vi "Tutorial_7_ICP_IP_save_table.vi"() -> ()   [LabVIEW 2020]
uses:
  <vilib>/Utility/file.llb/Write Delimited Spreadsheet (string).vi
  <vilib>/Utility/file.llb/Read Delimited Spreadsheet (string).vi
  <vilib>/regexp/Match Regular Expression.xnode
panel:
  out "data out":string
  out "ArraySize":i32
  out "subarray":string[](array[string])
  out "Login Details":string
  out "error out":errorcluster
  in  "file path (dialog if empty)":path
  in  "Registration UI":enum32{"Page 1", "Page 2"}(tab)
  in  "OK Button":bool
  in  "tbl Registration":string[][](table)
  in  "Login UI":enum32{"Page 1"}(tab)
  out "Status":bool
  in  "btnLogin":bool
  in  "Password":string
  in  "User Name":string
  # "Client"
  # "Server"
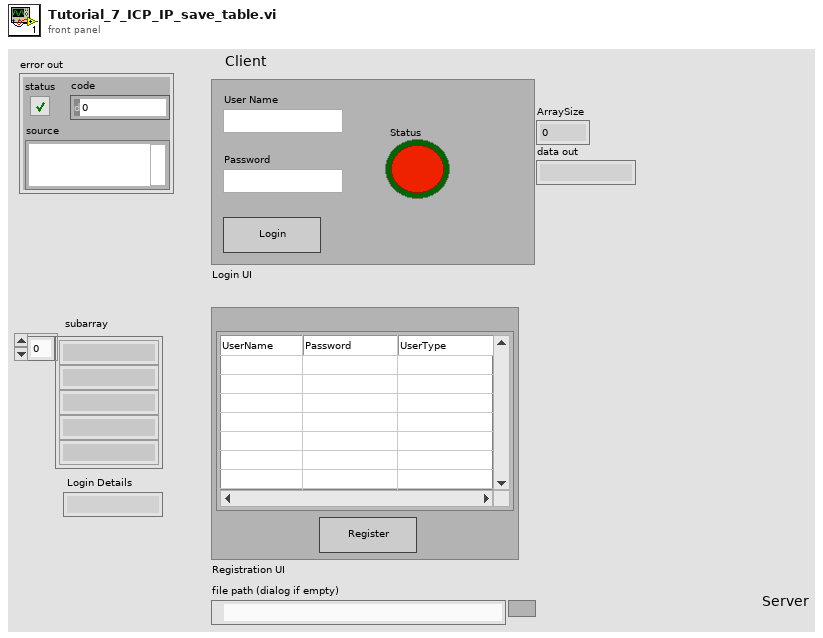
[diagram p1: front panel]
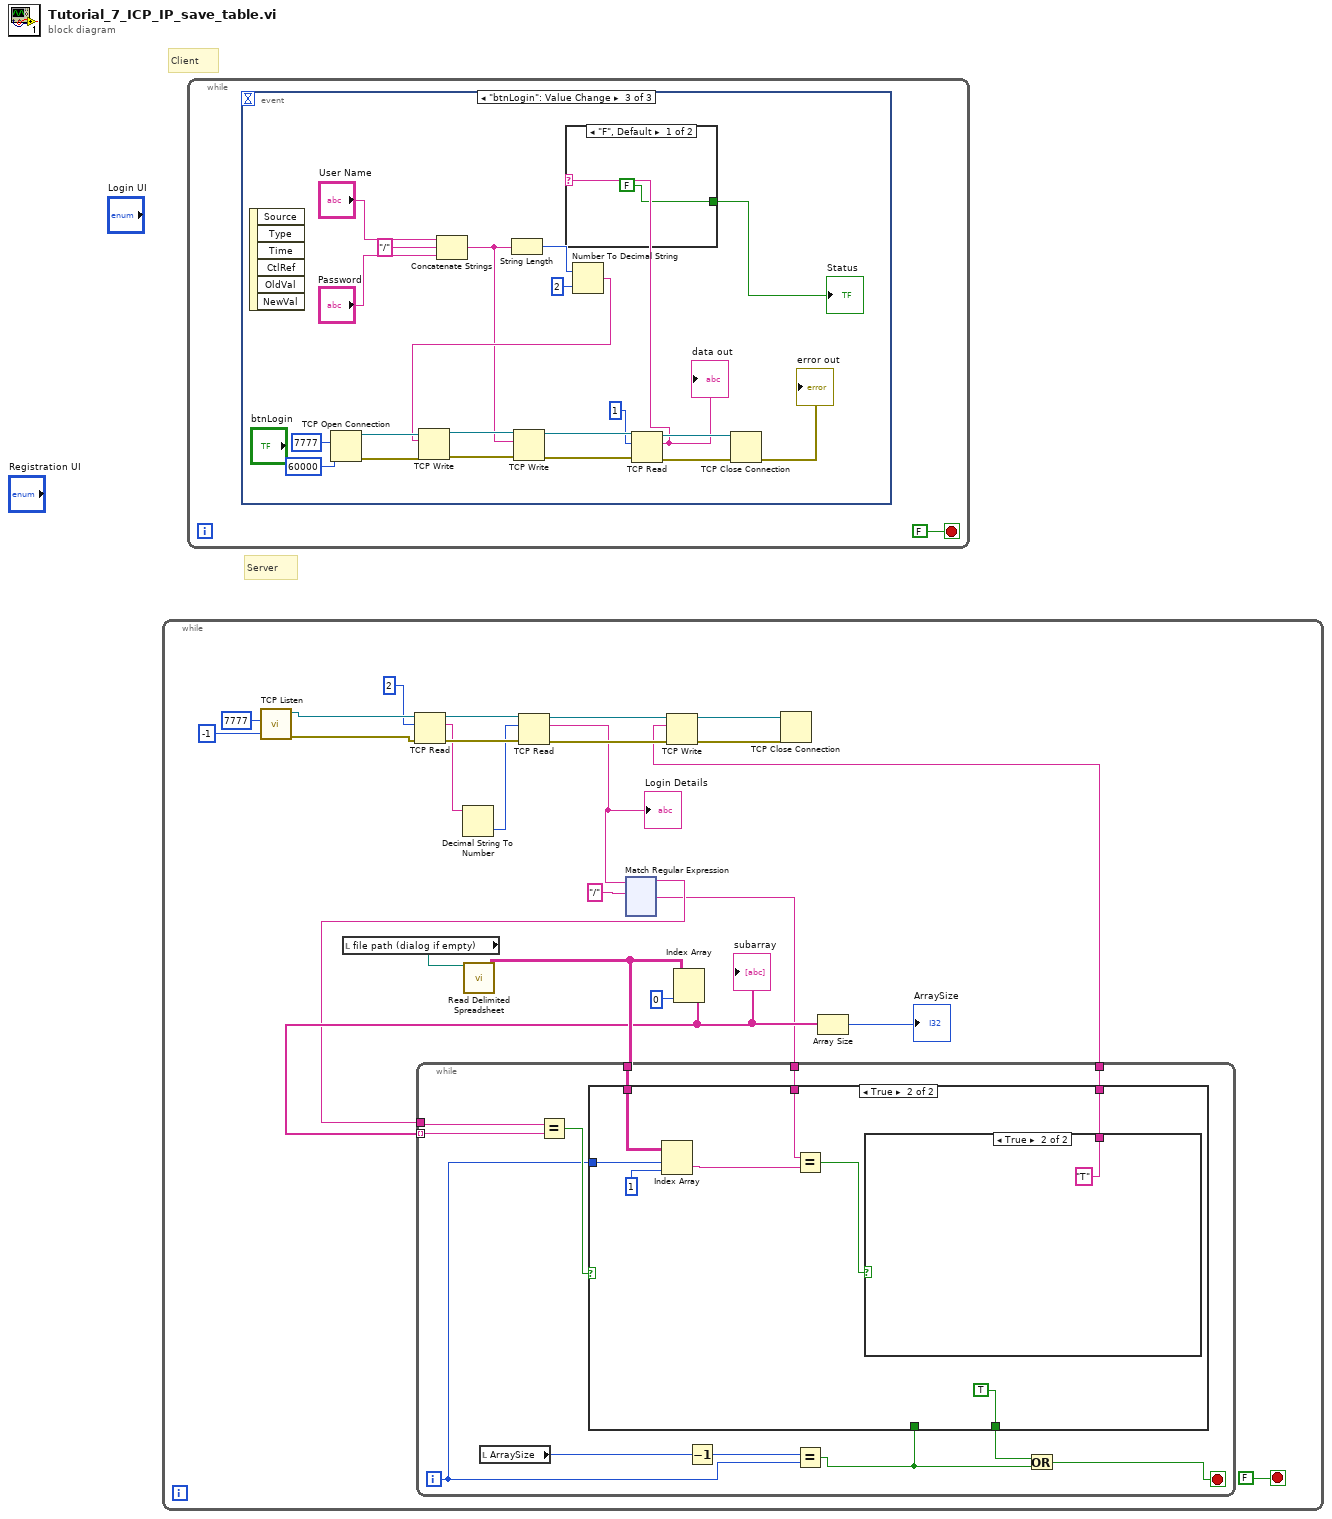
[diagram p0: block diagram]
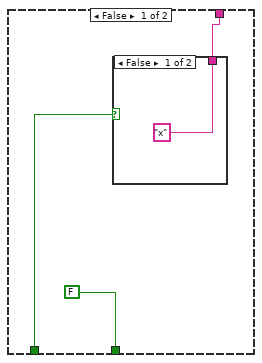
[diagram p2: hidden frame]
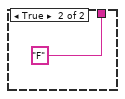
[diagram p3: hidden frame]
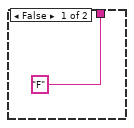
[diagram p4: hidden frame]
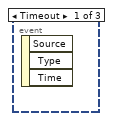
[diagram p5: hidden frame]
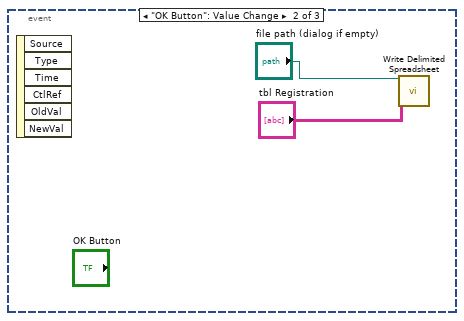
[diagram p6: hidden frame]
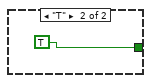
[diagram p7: hidden frame]
diagram:
  # "Server"
  # "Client"
  n1 = while {
    stop <- FALSE stop-if-true
    n2 = call <vilib>:"TCP Listen.vi"("timeout ms (wait forever: -1)"=-1, "port"=u16 7777) -> ("error out"=w17:errorcluster, "connection ID"=w20:refnum<k5>)  [unwired: 5 in, 3 out]
    n3 = local read "file path (dialog if empty)"() -> (w8:path)
    n4 = TCP Read(connection ID=w20, bytes to read=2, error in (no error)=w17) -> (connection ID out=w19:refnum<k5>, data out=w15:string, error out=w18:errorcluster)  [unwired: 2 in]
    n5 = Decimal String To Number(string=w15) -> (number=w14:i32)  [unwired: 2 in, 1 out]
    n6 = call-poly <vilib>:"Read Delimited Spreadsheet.vi"("file path (dialog if empty)"=w8) -> ("all rows"=w7:string[][])  [unwired: 9 in, 5 out]
    n7 = TCP Read(connection ID=w19, bytes to read=w14, error in (no error)=w18) -> (connection ID out=w21:refnum<k5>, data out=w10:string, error out=w24:errorcluster)  [unwired: 2 in]
    "Login Details" <- w10
    n8 = xnode "Match Regular Expression"("input string"=w10, "regular expression"="/") -> ("before match"=w3:string, "after match"=w2:string)  [unwired: 4 in, 3 out]
    n9 = Index Array "Index Array"(array=w7, index (col)=0 ("disabled index (col)")) -> (element=w5:string[])  [unwired: 1 in]
    "subarray" <- w5
    n10 = while {
      tunnel: w5 -> [w36] mode=indexing
      tunnel: w7 -> [w34]
      tunnel: [w33] -> w6
      tunnel: w3 -> [w26]
      tunnel: w2 -> [w25]
      i -> [w30]
      stop <- w29 stop-if-true
      n11 = local read "ArraySize"() -> (w32:i32)
      n12 = Equal?(x=w26, y=w36) -> (x = y?=w35:bool)
      n13 = Decrement(x=w32) -> (x-1=w31:i32)
      n14 = Equal?(x=w31, y=w30) -> (x = y?=w27:bool)
      n15 = case shown="True" w35 {
        tunnel: w34 -> [_ w49]
        tunnel: w30 -> [_ w47]
        tunnel: [w37 w44] -> w33
        tunnel: [FALSE TRUE] -> w28
        tunnel: w27 -> [w38 _]
        tunnel: w25 -> [_ w42]
        frame False {
          n16 = case shown="False" w38 {
            tunnel: ["x" "F"] -> w37
            frame False {
            }
            frame True {
            }
          }
        }
        frame True {
          n17 = Index Array(array=w49, index (row)=w47, index (col)=1 ("disabled index (col)")) -> (element=w46:string)
          n18 = Equal?(x=w42, y=w46) -> (x = y?=w45:bool)
          n19 = case shown="True" w45 {
            tunnel: ["F" "T"] -> w44
            frame False {
            }
            frame True {
            }
          }
        }
      }
      n20 = Or(x=w28, y=w27) -> (x .or. y?=w29:bool)
    }
    n21 = TCP Write(connection ID=w21, data in=w6, error in (no error)=w24) -> (connection ID out=w22:refnum<k5>, error out=w23:errorcluster)  [unwired: 1 in, 1 out]
    n22 = TCP Close Connection(connection ID=w22, error in (no error)=w23) -> ()  [unwired: 1 in, 2 out]
    n23 = Array Size(array=w5) -> (size(s)=→"ArraySize":i32)
  }
  n24 = while {
    stop <- FALSE stop-if-true
    n25 = event shown="[2] \"btnLogin\": Value Change" {
      selector: _ -> [_ _ _]
      dyn-events: _ -> [_ _ _]
      timeout: _ -> [_ _ _]
      event Timeout {
        n26 = event-data() -> ()  [unwired: 1 in, 3 out]
      }
      event "OK Button": Value Change {
        n27 = event-data() -> ()  [unwired: 1 in, 6 out]
        n28 = call-poly <vilib>:"Write Delimited Spreadsheet.vi"("file path (dialog if empty)"="file path (dialog if empty)", "2D data"="tbl Registration") -> ()  [unwired: 12 in, 2 out]
      }
      event "btnLogin": Value Change {
        n29 = event-data() -> ()  [unwired: 1 in, 6 out]
        n30 = TCP Open Connection(remote port or service name=u16 7777, timeout ms (60000)=60000) -> (connection ID=w187:refnum<k5>, error out=w185:errorcluster)  [unwired: 3 in]
        n31 = Concatenate Strings "Concatenate Strings"("User Name", "/" ("string"), "Password") -> (w174:string)
        n32 = String Length(string=w174) -> (length=w177:i32)
        n33 = Number To Decimal String(number=w177, width (-)=i16 2) -> (decimal integer string=w175:string)
        n34 = TCP Write(connection ID=w187, data in=w175, error in (no error)=w185) -> (connection ID out=w186:refnum<k5>, error out=w184:errorcluster)  [unwired: 1 in, 1 out]
        n35 = TCP Write(connection ID=w186, data in=w174, error in (no error)=w184) -> (connection ID out=w189:refnum<k5>, error out=w188:errorcluster)  [unwired: 1 in, 1 out]
        n36 = TCP Read(connection ID=w189, bytes to read=1, error in (no error)=w188) -> (connection ID out=w182:refnum<k5>, data out=w172:string, error out=w183:errorcluster)  [unwired: 2 in]
        "data out" <- w172
        n37 = case shown="\"F\", Default" w172 {
          tunnel: [FALSE TRUE ("Status")] -> w171
          frame "F", Default {
          }
          frame "T" {
          }
        }
        "Status" <- w171
        n38 = TCP Close Connection(connection ID=w182, error in (no error)=w183) -> (error out=→"error out":errorcluster)  [unwired: 1 in, 1 out]
      }
    }
  }
